vi "Execute Command.vi"(8 "error in (no error)":errorcluster, 10 "UI Load SubPanel Display in":refnum<class "UI Load SubPanel Display.lvclass">, 11 "User Interface References":T1={"This VI"=refnum, "User Interace Plugin"=refnum, "UI Picture Container References"={"Header Image"=refnum, "Footer Image"=refnum}, "Sliding Menu XControl"=refnum, "Menu Container"=refnum, "UI Configuration Information"={"Space Between Buttons"=3, "Number of Buttons to Show"=6, "Header Image"=path "Images/Blue Background.bmp", "Footer Image"=path "Images/Blue Background.bmp"}, "Header Text"=refnum}) -> (0 "error out":errorcluster, 1 "Stop?":bool, 2 "UI Load SubPanel Display out":refnum<class "UI Load SubPanel Display.lvclass">, 3 "User Interface References Out":T1={"This VI"=refnum, "User Interace Plugin"=refnum, "UI Picture Container References"={"Header Image"=refnum, "Footer Image"=refnum}, "Sliding Menu XControl"=refnum, "Menu Container"=refnum, "UI Configuration Information"={"Space Between Buttons"=3, "Number of Buttons to Show"=6, "Header Image"=path "Images/Blue Background.bmp", "Footer Image"=path "Images/Blue Background.bmp"}, "Header Text"=refnum})   [LabVIEW 2011, in "UI Load SubPanel Display.lvclass"]
uses:
  UI Load SubPanel Display.lvclass
  Main Type Definitions/User Interface Type Definitions.ctl
  Main Type Definitions/UI Picture Containers.ctl
  Sliding Menu/Sliding Menu Library/Sliding Menu xControl/Sliding Menu XControl.xctl
  UI Control Definitions/UI Configuration Information.ctl
  UI Slide Panel On Screen/Slide Panel On Screen.lvclass
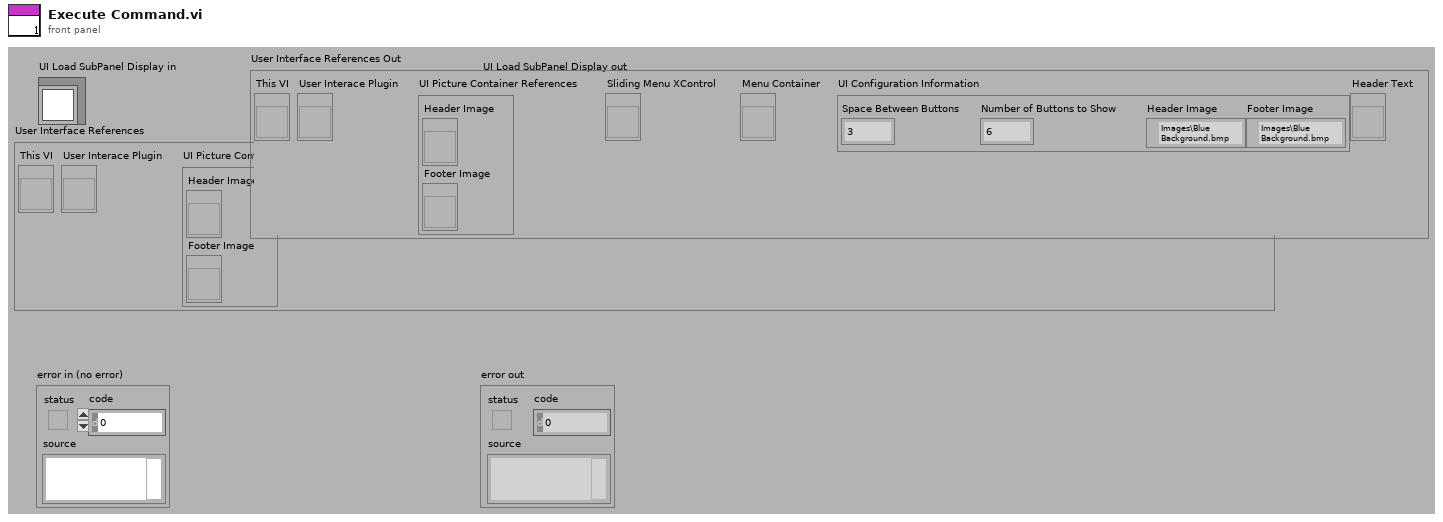
[diagram p1: front panel]
types:
  T1 = typedef "User Interface Type Definitions.ctl" = cluster{"This VI":refnum<vi>, "User Interace Plugin":refnum<vi>, "UI Picture Container References":T2, "Sliding Menu XControl":refnum<vi>, "Menu Container":refnum<vi>, "UI Configuration Information":T3, "Header Text":refnum<vi>}
  T2 = typedef "UI Picture Containers.ctl" = cluster{"Header Image":refnum<vi>, "Footer Image":refnum<vi>}
  T3 = typedef "UI Configuration Information.ctl" = cluster{"Space Between Buttons":i32, "Number of Buttons to Show":i32, "Header Image":path, "Footer Image":path}
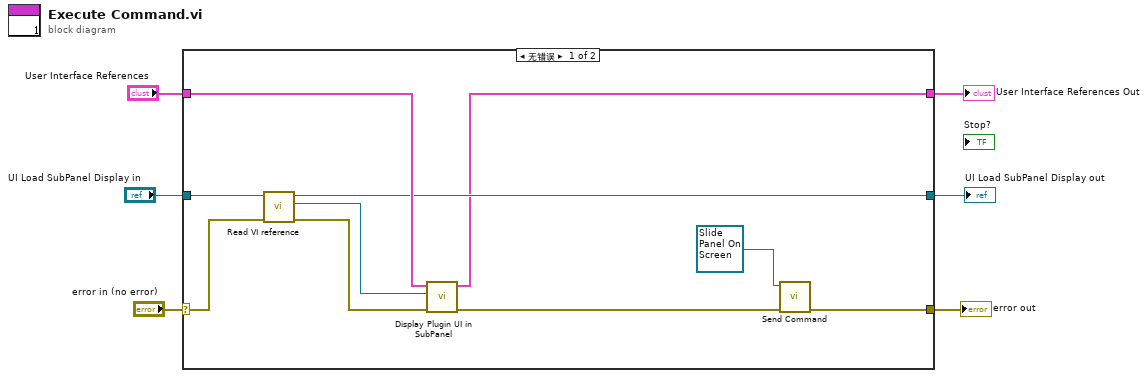
[diagram p0: block diagram]
diagram:
  n1 = case shown="无错误" "error in (no error)" {
    selector: "error in (no error)" -> [w11 w17]
    tunnel: "User Interface References" -> [w16 w19]
    tunnel: "UI Load SubPanel Display in" -> [w14 w18]
    tunnel: [w13 w18] -> w4
    tunnel: [w8 w17] -> w3
    tunnel: [w7 w19] -> w2
    frame No Error {
      n2 = call-dynamic "Read VI reference.vi"("error in (no error)"=w11, "UI Load SubPanel Display in"=w14) -> ("error out"=w12:errorcluster, "VI reference"=w15:refnum<vi>, "UI Load SubPanel Display out"=w13:refnum<class "UI Load SubPanel Display.lvclass">)  [unwired: 7 in]
      n3 = call "Display Plugin UI in SubPanel.vi"("error IO"=w12, "VI reference"=w15, "User Interface References"=w16) -> ("error out"=w9:errorcluster, "User Interface References Out"=w7:T1)  [unwired: 7 in]
      n4 = call-dynamic "Send Command.vi"("error in (no error)"=w9, "UI Command Manager in"=refnum<class "Slide Panel On Screen.lvclass"> refnum ("Slide Panel On Screen.lvclass")) -> ("error out"=w8:errorcluster)  [unwired: 8 in, 1 out]
    }
    frame Error {
    }
  }
  "error out" <- w3
  "UI Load SubPanel Display out" <- w4
  "User Interface References Out" <- w2
